vi "DashboardMain.vi"() -> ()   [LabVIEW 2014]
uses:
  RobotToDashboardCluster.ctl
  DashboardToRobotCluster.ctl
panel:
  out "Totes In Robot":bool[](array[boolean])
  out "Air Pressure":dbl(slide) scale=0.0..100.0
  out "Heading":dbl(knob) scale=0.0..360.0
  out "Attempting to Connect":bool
  out "Connected":bool
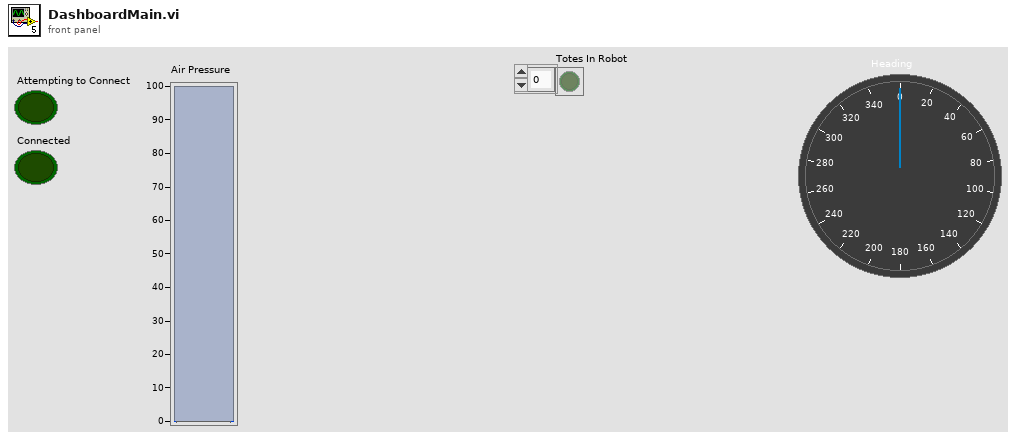
[diagram p1: front panel]
types:
  T1 = typedef "DashboardToRobotCluster.ctl" = cluster{"Test":dbl}
  T2 = typedef "RobotToDashboardCluster.ctl" = cluster{"Front Right Motor":dbl, "Front Left Motor":dbl, "Rear Right Motor":dbl, "Rear Left Motor":dbl, "Current Heading":dbl, "Can Grabber Closed":bool, "Last Can Grabber Position":enum16{"Floor", "Level 1", "Level 2", "Level 3", "Level 4", "Level 5", "Level 6"}, "Can Grabber Movement":enum16{"At Rest", "Moving Up", "Moving Down"}, "Tote lift Up":bool, "Primary Feeder running":bool, "Secondary Feeder running":bool, "Totes In Robot":dbl, "Pressure In Tank":dbl}
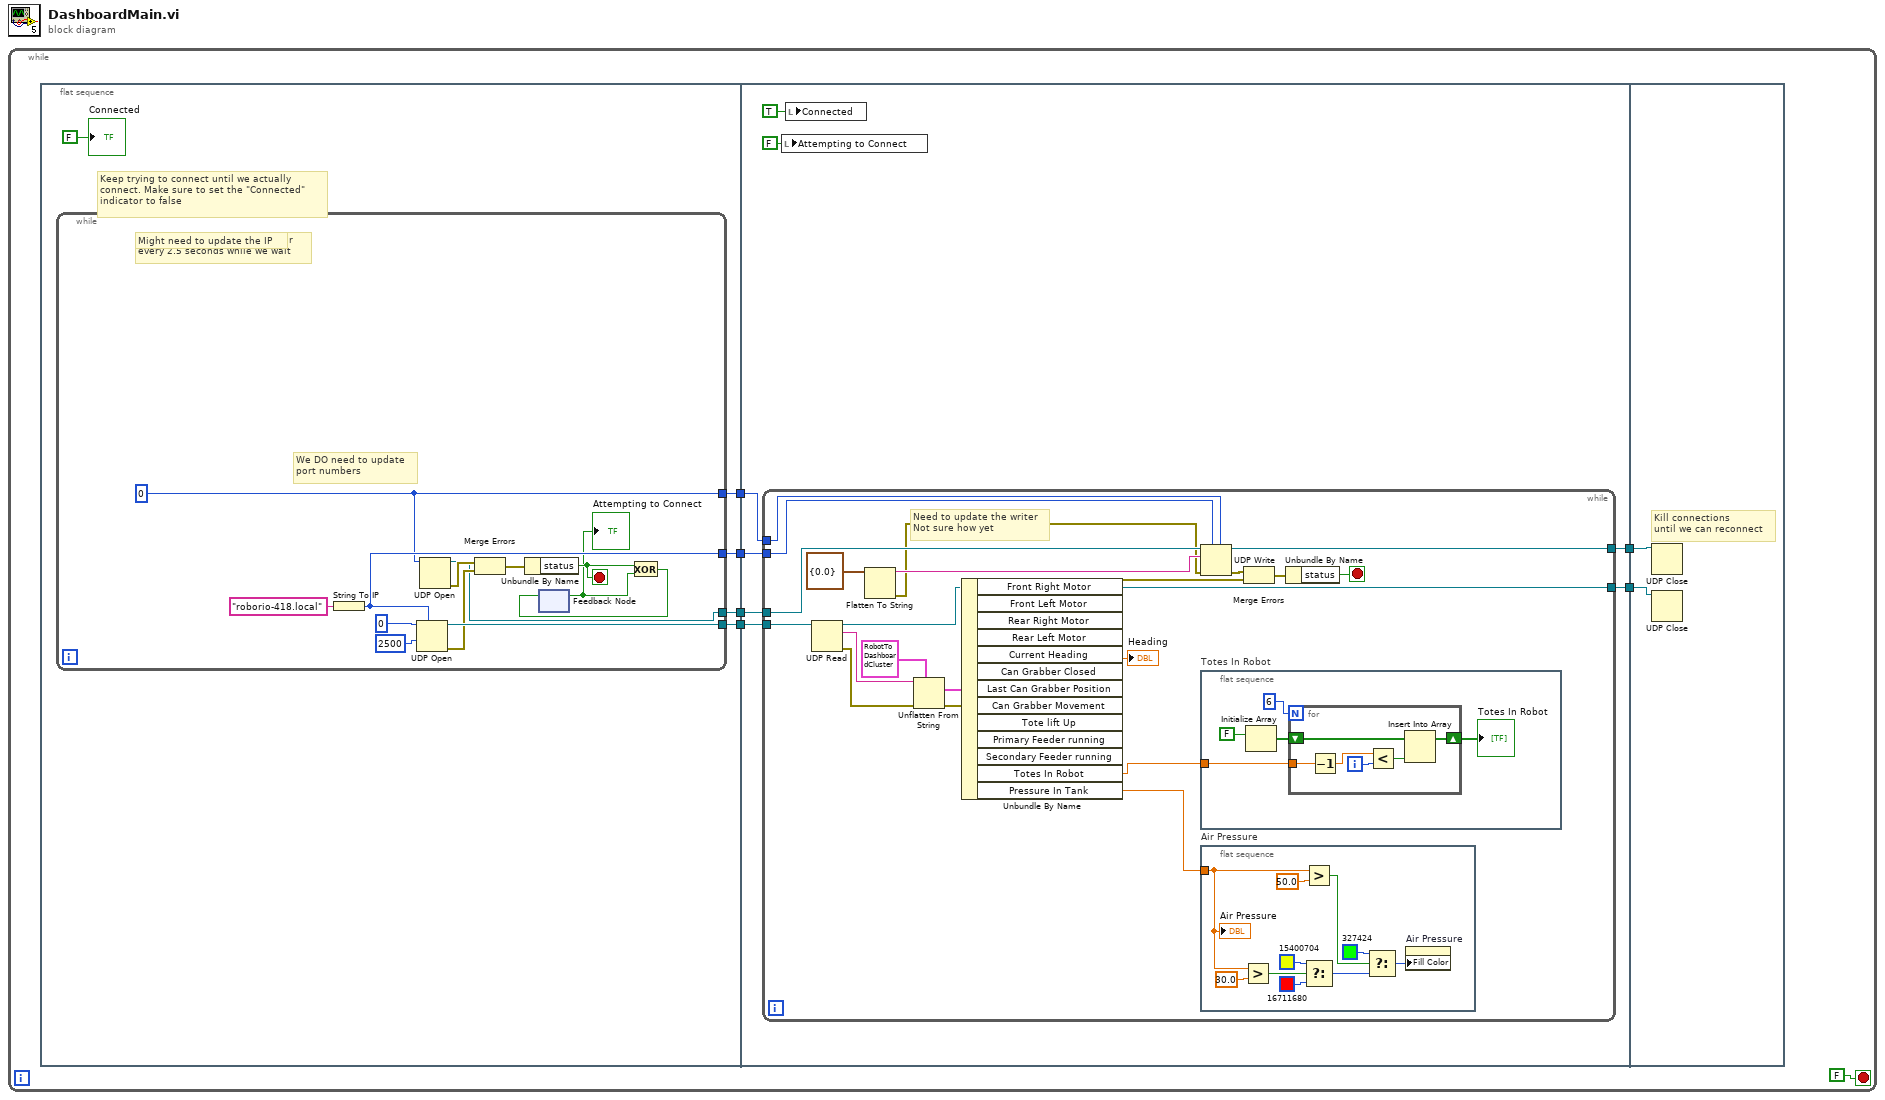
[diagram p0: block diagram]
diagram:
  n1 = while {
    stop <- FALSE stop-if-true
    n2 = flat-sequence {
      tunnel: [w12] -> w6
      tunnel: [w11] -> w5
      tunnel: [w10] -> w4
      tunnel: [w9] -> w3
      tunnel: w6 -> [w33]
      tunnel: w5 -> [w31]
      tunnel: w4 -> [w30]
      tunnel: w3 -> [w29]
      tunnel: [w27] -> w2
      tunnel: [w26] -> w1
      tunnel: w2 -> [w76]
      tunnel: w1 -> [w75]
      frame #0 {
        # "Keep trying to connect until we actually\nconnect. Make sure to set the \"Connected\"\nindicator to false"
        n3 = while {
          tunnel: [w20] -> w12
          tunnel: [w16] -> w11
          tunnel: [w15] -> w10
          tunnel: [w14] -> w9
          stop <- w21 stop-if-true
          w14 = u16 0 ("port")
          # "We DO need to update\nport numbers"
          # "Might need to update the IP"
          # "Flash the \"Connecting\" indicator\nevery 2.5 seconds while we wait"
          n4 = String To IP(1:"roborio-418.local" ("name")) -> (0:w15:u32)
          n5 = UDP Open(7:w15, 9:2500 ("timeout ms (25000)"), 11:u16 0 ("port")) -> (port=w20:refnum<k16>, 0:w18:errorcluster)  [unwired: 2 in, 1 out]
          n6 = UDP Open(11:w14) -> (port=w16:refnum<k16>, 0:w19:errorcluster)  [unwired: 4 in, 1 out]
          n7 = Merge Errors(w19, w18) -> (w17:errorcluster)
          n8 = Unbundle By Name(w17) -> ("status"=w21:bool)
          n9 = feedback #1() -> (w13:bool)  [unwired: 1 in]
          "Attempting to Connect" <- w13
          n10 = Exclusive Or(1:w13, 2:w21) -> (0:w22:bool)
          n11 = feedback-in #1(w22) -> ()
        }
        "Connected" <- FALSE ("Communications")
      }
      frame #1 {
        n12 = while {
          tunnel: w33 -> [w48]
          tunnel: w31 -> [w47]
          tunnel: w30 -> [w46]
          tunnel: w29 -> [w45]
          tunnel: [w39] -> w27
          tunnel: [w38] -> w26
          stop <- w51 stop-if-true
          # "Need to update the writer\nNot sure how yet"
          n13 = UDP Read(connection ID=w48) -> (data out=w53:string, error out=w52:errorcluster, 3:w38:refnum<k16>)  [unwired: 3 in, 2 out]
          n14 = Flatten To String(anything=T1 {"Test"=0.0} ("Cluster")) -> (data string=w44:string, error out=w43:errorcluster)  [unwired: 3 in, 1 out]
          n15 = Unflatten From String(type=T2 {"Front Right Motor"=0.0, "Front Left Motor"=0.0, "Rear Right Motor"=0.0, "Rear Left Motor"=0.0, "Current Heading"=0.0, "Can Grabber Closed"=FALSE, "Last Can Grabber Position"=enum."Floor", "Can Grabber Movement"=enum."At Rest", "Tote lift Up"=FALSE, "Primary Feeder running"=FALSE, "Secondary Feeder running"=FALSE, "Totes In Robot"=0.0, "Pressure In Tank"=0.0} ("Dashboard Cluster"), binary string=w53, error in (no error)=w52) -> (value=w49:T2, error out=w41:errorcluster)  [unwired: 2 in, 1 out]
          n16 = Unbundle By Name(w49) -> ("Current Heading"=→"Heading":dbl, "Totes In Robot"=w34:dbl, "Pressure In Tank"=w35:dbl)  [unwired: 10 out]
          n17 = UDP Write(address=w46, port or service name=w45, connection ID=w47, data in=w44, 8:w43) -> (error out=w42:errorcluster, 3:w39:refnum<k16>)  [unwired: 1 in]
          n18 = flat-sequence "Totes In Robot" {
            tunnel: w34 -> [w65]
            frame #0 {
              n19 = Initialize Array(FALSE) -> (w67:bool[])  [unwired: 1 in]
              n20 = for {
                N: 6 -> [_]
                shift-right: [w73] -> w64
                shift-left: w67 -> [w74]
                tunnel: w65 -> [w72]
                i -> [w69]
                n21 = Decrement(x=w72) -> (x-1=w70:dbl)
                n22 = Less?(x=w70, y=w69) -> (x < y?=w71:bool)
                n23 = Insert Into Array(array=w74, new element=w71) -> (w73:bool[])  [unwired: 1 in]
              }
              "Totes In Robot" <- w64
            }
          }
          n24 = flat-sequence "Air Pressure" {
            tunnel: w35 -> [w56]
            frame #0 {
              n25 = Greater?(x=w56, y=30.0) -> (0:w57:bool)
              n26 = Greater?(x=w56, y=50.0) -> (0:w62:bool)
              n27 = Select(t=u32 15400704, s=w57, f=u32 16711680) -> (s? t:f=w59:u32)
              n28 = Select(t=u32 327424, s=w62, f=w59) -> (s? t:f=w60:u32)
              n29 = property on="Air Pressure" class="Slide (strict)"("Fill Color"=w60) -> ()  [unwired: 2 in, 2 out]
              "Air Pressure" <- w56
            }
          }
          n30 = Merge Errors(w42, w41) -> (w40:errorcluster)
          n31 = Unbundle By Name(w40) -> ("status"=w51:bool)
        }
        n32 = local write "Attempting to Connect"(FALSE ("Connecting")) -> ()
        n33 = local write "Connected"(TRUE ("Connected")) -> ()
      }
      frame #2 {
        # "Kill connections\nuntil we can reconnect"
        n34 = UDP Close(connection ID=w76) -> ()  [unwired: 1 in, 2 out]
        n35 = UDP Close(connection ID=w75) -> ()  [unwired: 1 in, 2 out]
      }
    }
  }
